vi "Calc max speed at certain distance.vi"(8 "error in (no error)":errorcluster, 11 "Distance from dest":dbl=500.0) -> (0 "error out":errorcluster, 3 "Speed":dbl)   [LabVIEW 2016]
panel:
  in  "Min dist for movement":dbl=50.0
  in  "min speed":dbl=0.3
  in  "Distance at speed 4":dbl=300.0
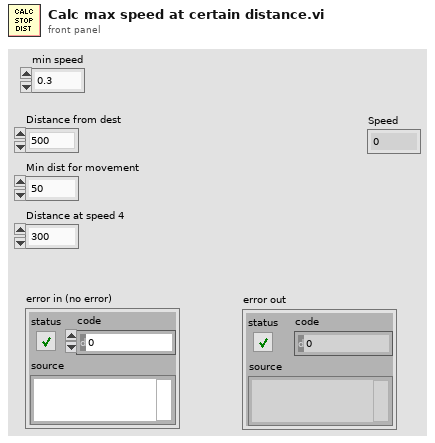
[diagram p1: front panel]
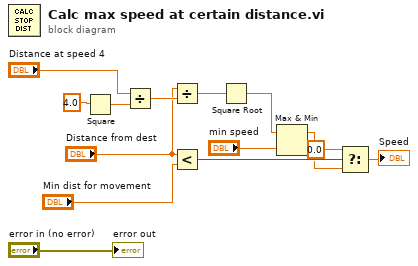
[diagram p0: block diagram]
diagram:
  n1 = Square(x=4.0) -> (x^2=w13:dbl)
  n2 = Divide(x="Distance at speed 4", y=w13) -> (x/y=w10:dbl)
  n3 = Divide(x="Distance from dest", y=w10) -> (x/y=w9:dbl)
  n4 = Less?(x="Distance from dest", y="Min dist for movement") -> (x < y?=w4:bool)
  n5 = Square Root(x=w9) -> (sqrt(x)=w8:dbl)
  n6 = Max & Min(x=w8, y="min speed") -> (max(x,y)=w2:dbl)  [unwired: 1 out]
  n7 = Select(t=0.0, s=w4, f=w2) -> (s? t:f=→"Speed":dbl)
  "error out" <- "error in (no error)"
